vi "Save S2P - SParam.vi"(8 "error in":errorcluster, 10 "SnP File Path":path, 11 "Refnum in":refnum<k21>) -> (0 "error out":errorcluster, 3 "Refnum out":refnum<k21>)   [LabVIEW 2023]
uses:
  <resource>/objmgr/RFmxVNA.rc
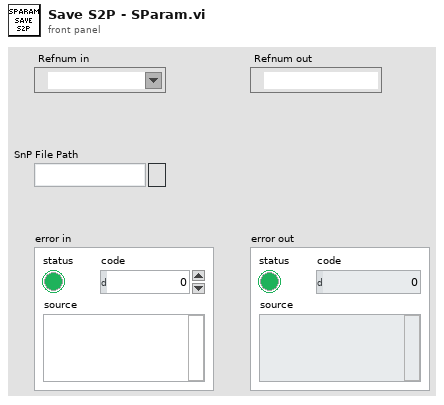
[diagram p1: front panel]
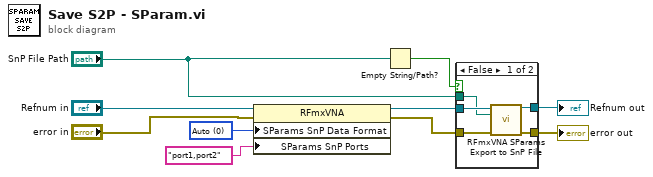
[diagram p0: block diagram]
diagram:
  w5 = 0 items=["Auto", "Log Magnitude-Angle", "Real-Imaginary", "Linear Magnitude-Angle"] ("SParams SnP Data Format")
  n1 = property class="RFmxVNA"(reference="Refnum in", error in="error in", "SParams SnP Data Format"=w5, "SParams SnP Ports"="port1,port2") -> (reference out=w3:refnum<k21>, error out=w4:errorcluster)
  n2 = Empty String/Path?(string/path="SnP File Path") -> (empty?=w9:bool)
  n3 = case shown="False" w9 {
    tunnel: [w15 w17] -> w1
    tunnel: [w14 w16] -> w2
    tunnel: w3 -> [w13 w17]
    tunnel: w4 -> [w12 w16]
    tunnel: "SnP File Path" -> [w11 _]
    frame False {
      n4 = call <vilib>:"RFmxVNA SParams Export to SnP File.vi"("Instrument Handle In"=w13, "SnP File Path"=w11, "error in (no error)"=w12) -> ("Instrument Handle Out"=w15:refnum<k21>, "error out"=w14:errorcluster)  [unwired: 11 in]
    }
    frame True {
    }
  }
  "error out" <- w2
  "Refnum out" <- w1
